vi "Array to Plot 2016.vi"(8 "Input Cumulative Array":dbl[][](array[numeric]) format="%.2f", 9 "Input Real Time Array":dbl[][](array[numeric]) format="%.2f") -> (0 "Cumulative - Depth vs.Drive Rate":cluster{dbl[], dbl[]} {"?" format="%.2f"; "?" format="%.2f"}, 1 "Cumulative - Depth vs. Ik":cluster{dbl[], dbl[]} {"?" format="%.2f"; "?" format="%.2f"}, 2 "Real Time - Depth vs. Drive Rate":cluster{dbl[], dbl[]} {"?" format="%.2f"; "?" format="%.2f"}, 3 "Real Time - Depth vs. Ik":cluster{dbl[], dbl[]} {"?" format="%.2f"; "?" format="%.2f"}, 4 "Current Ik":dbl format="%.2f", 5 "Depth Rate":dbl format="%.2f")   [LabVIEW 2016]
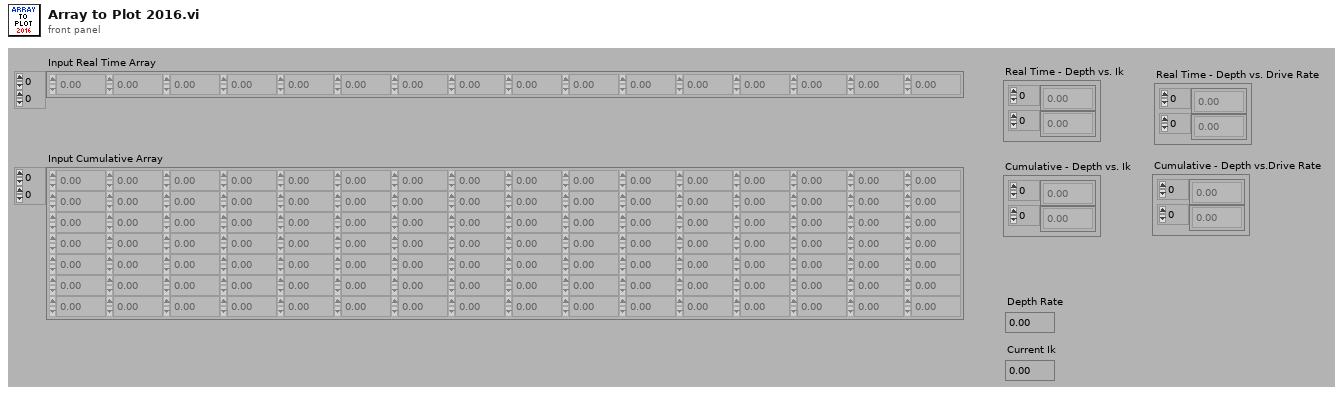
[diagram p1: front panel]
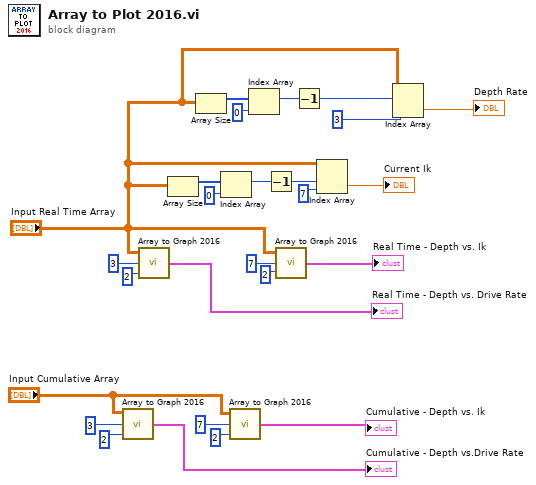
[diagram p0: block diagram]
diagram:
  n1 = call "Array to Graph 2016.vi"("Y Index"=2, "X Index"=3, "Input 2-D Array"="Input Cumulative Array") -> ("Output Cluster to Graph"=→"Cumulative - Depth vs.Drive Rate":cluster{dbl[], dbl[]})
  n2 = call "Array to Graph 2016.vi"("Y Index"=2, "X Index"=3, "Input 2-D Array"="Input Real Time Array") -> ("Output Cluster to Graph"=→"Real Time - Depth vs. Drive Rate":cluster{dbl[], dbl[]})
  n3 = Array Size(array="Input Real Time Array") -> (size(s)=w14:i32[])
  n4 = Array Size(array="Input Real Time Array") -> (size(s)=w7:i32[])
  n5 = Index Array(array=w14, index=0) -> (element=w8:i32)
  n6 = call "Array to Graph 2016.vi"("Y Index"=2, "X Index"=7, "Input 2-D Array"="Input Cumulative Array") -> ("Output Cluster to Graph"=→"Cumulative - Depth vs. Ik":cluster{dbl[], dbl[]})
  n7 = Index Array(array=w7, index=0) -> (element=w5:i32)
  n8 = Decrement(x=w8) -> (x-1=w12:i32)
  n9 = call "Array to Graph 2016.vi"("Y Index"=2, "X Index"=7, "Input 2-D Array"="Input Real Time Array") -> ("Output Cluster to Graph"=→"Real Time - Depth vs. Ik":cluster{dbl[], dbl[]})
  n10 = Decrement(x=w5) -> (x-1=w3:i32)
  n11 = Index Array(array="Input Real Time Array", index (row)=w12, index (col)=7) -> (element=→"Current Ik":dbl)
  n12 = Index Array(array="Input Real Time Array", index (row)=w3, index (col)=3) -> (element=→"Depth Rate":dbl)
